vi "Actor Core.vi"(8 "error in":errorcluster, 11 "DUTMotor in":refnum<class "DUTMotor.lvclass">) -> (0 "error out":errorcluster, 3 "Actor out":refnum<class "Actor.lvclass">)   [LabVIEW 2024, in "DUTMotor Actor.lvlib" / "DUTMotor.lvclass"]
doc: "<p>(<strong>Filename</strong>: <span class=\"dnl\">Actor Framework.lvlib:Actor.lvclass:Actor Core.vi</span>)</p>\n<p>Receives messages to the actor, reacts to them, and initiates any error handling that may shut the actor down.</p>\n<p>Descendant classes may override this VI to append parallel tasks for the actor to complete while it handles messages. Overrides use the <a href=\"nihelplauncher://docs/csh?context=lvcore_glang_udclass\">Call Parent Class Method</a> node.</p>"
uses:
  DUTMotor.lvclass
  C:/Program Files (x86)/National Instruments/LabVIEW 2024/vi.lib/ActorFramework/Actor/Actor.lvclass
  <vilib>/ActorFramework/Actor/Actor.lvclass
  DUTMotor.lvclass/DUTMotor.ctl
  DUTMotorActFunc.ctl
  <vilib>/ActorFramework/Actor/Actor.lvclass/Actor.ctl
  MFActor/ActorMessage/MF Task Name.ctl
  MFActor/NestedActorName.ctl
  MFActor/DeviceAlias.ctl
  ref/PCANUSB/PCANUSB.lvclass
  MFActor/ActorMessage/MFActorMsg.lvclass
panel:
  out "UpdateData":bool
  out "Col Index Map":map{string, i32}(c390)
  out "MeasData":dbl[](array[numeric])
  out "In Query":bool
  out "Data":u8[](array[numeric])
  in  "EndProc":bool
  out "Connected":bool
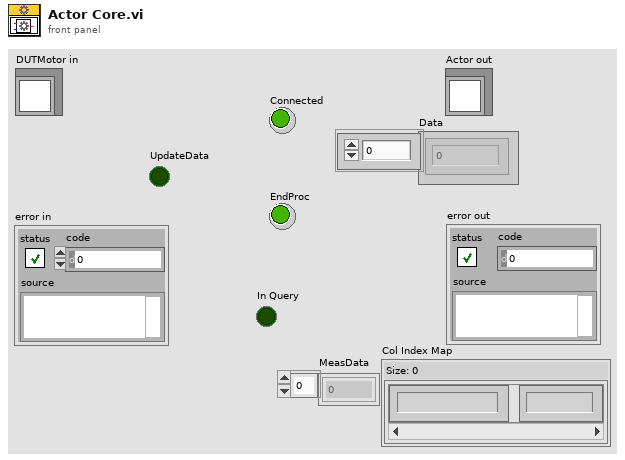
[diagram p1: front panel]
types:
  T1 = typedef "DUTMotorActFunc.ctl" = enum16{"None", "Config", "ConfigMeasData", "Query", "ConvertData", "End"}
  T2 = typedef "NestedActorName.ctl" = enum16{"None", "4503#0", "4503#1", "AIO#0", "AIO#1", "DIO", "PID", "TCPIP", "TestAngle", "TestFixPt", "TestMultiPt", "TestSinWave", "PW3390", "ADAM4118", "DUT Motor"}
  T3 = typedef "MF Task Name.ctl" = enum16{"DIChanged", "UpdateErrorCode", "SetTorque", "SetDriveTorque", "DataUpdated", "RunningTestProc", "StreamCtrl", "RunPID", "StopTest", "TCP Conn", "RefreshAutoUI", "ZeroAngle", "NestedActorLaunched", "NestedActorEnded", "ShowPsMsg"}
  T4 = typedef "DeviceAlias.ctl" = enum16{"TQM0", "TQM1", "PM", "THERMO", "DC POWER", "DUT Motor"}
  T5 = cluster{"message_id":i32, "CAN Signals":cluster{"signal_name":string, "start_bit":i32, "length":i32, "byte_order":string, "sign":string, "factor":dbl, "offset":dbl, "unit":string}[]}[]
  T6 = cluster{"message_id":i32, "CAN Signals":cluster{"signal_name":string, "start_bit":i32, "length":i32, "byte_order":string, "sign":string, "factor":dbl, "offset":dbl, "unit":string}[]}
  T7 = cluster{"signal_name":string, "start_bit":i32, "length":i32, "byte_order":string, "sign":string, "factor":dbl, "offset":dbl, "unit":string}[]
  T8 = cluster{"MF Msg Enum":T3, cluster{"MeasData":dbl[], "Device":T4}}
  T9 = cluster{"DUTMotorActFunc":T1, "ConfigMeasData":string[]}
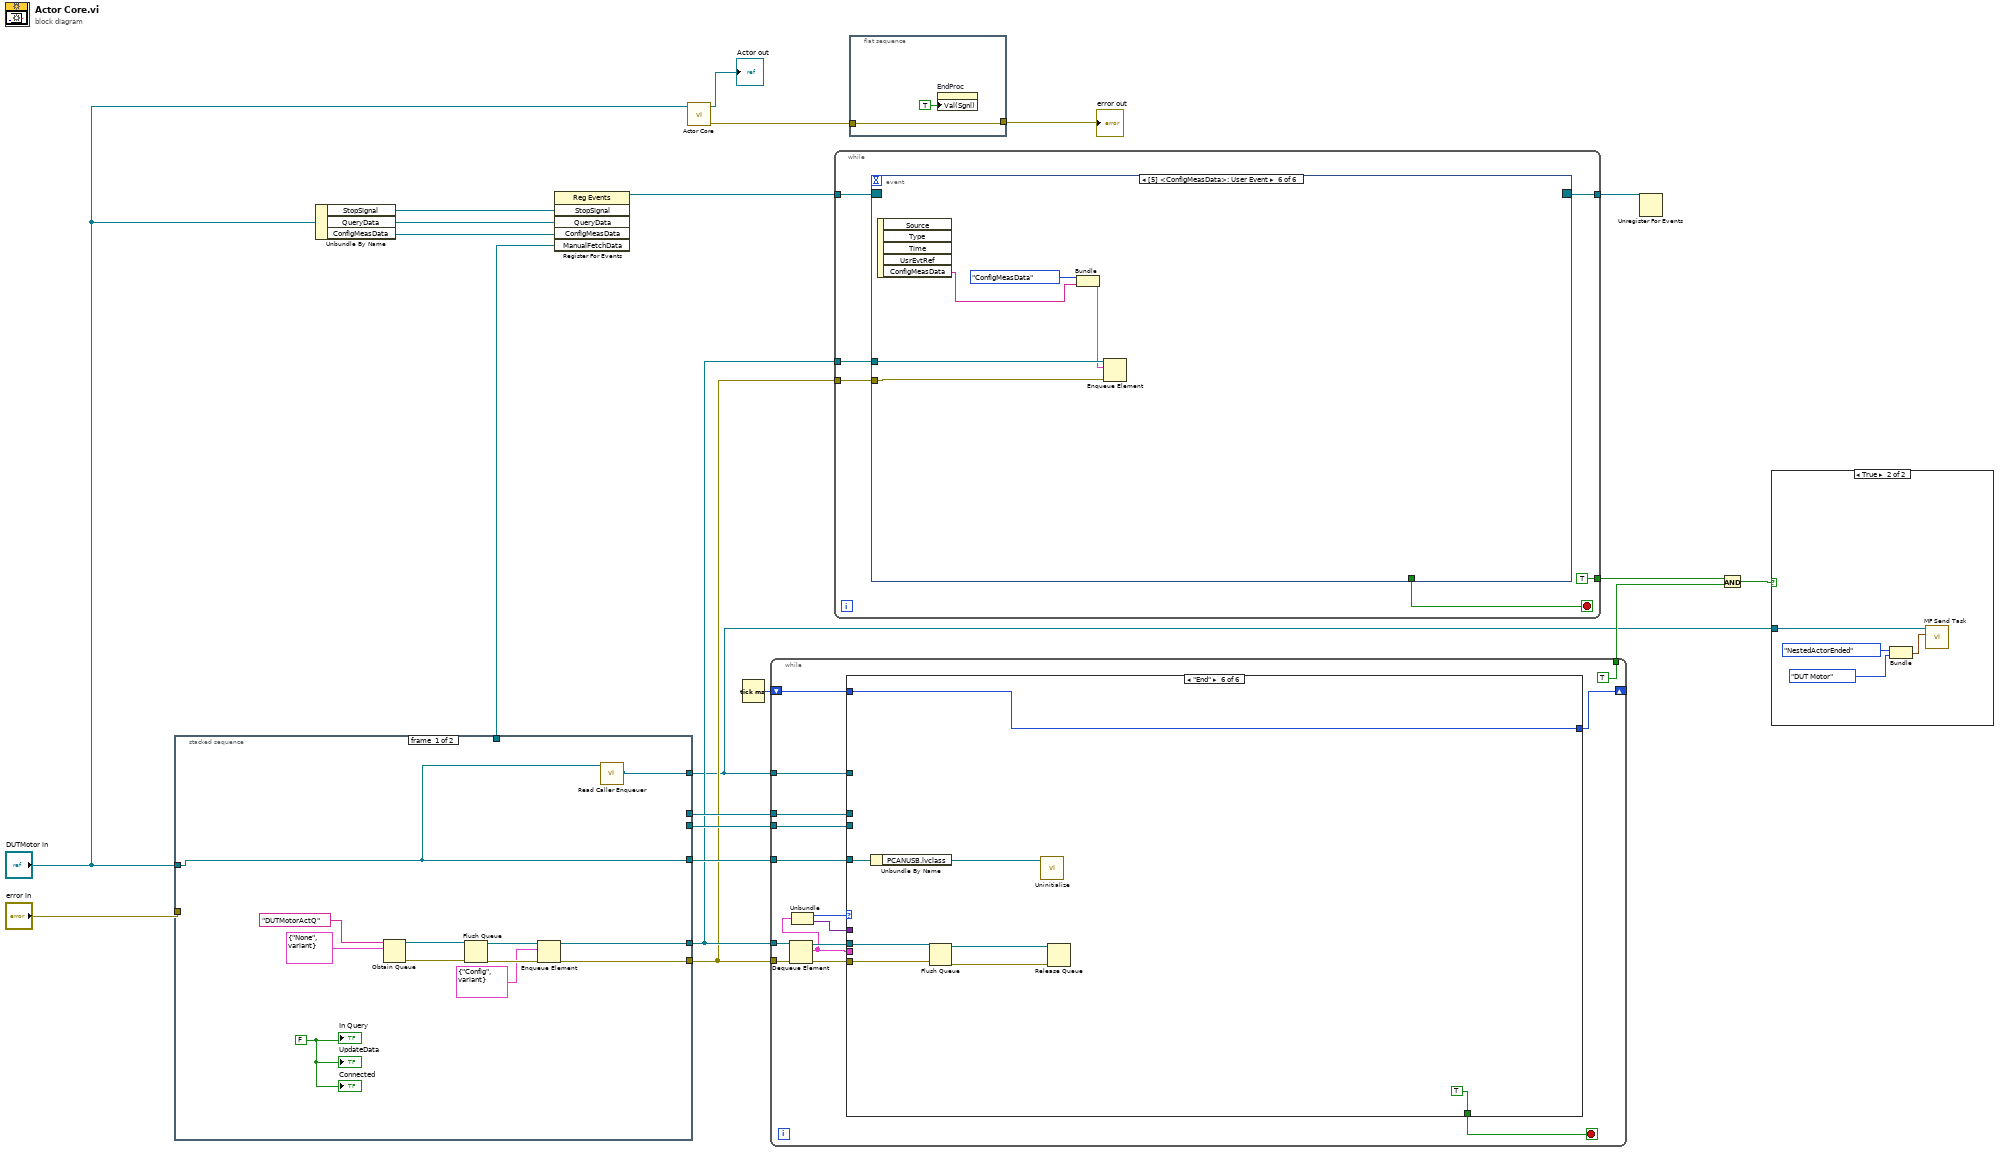
[diagram p0: block diagram]
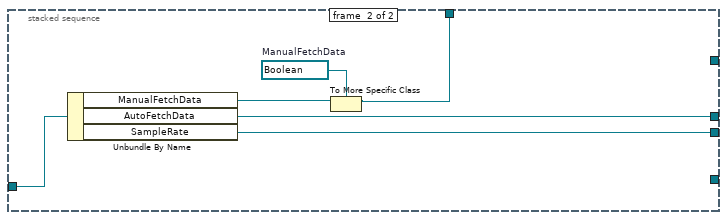
[diagram p3: hidden frame]
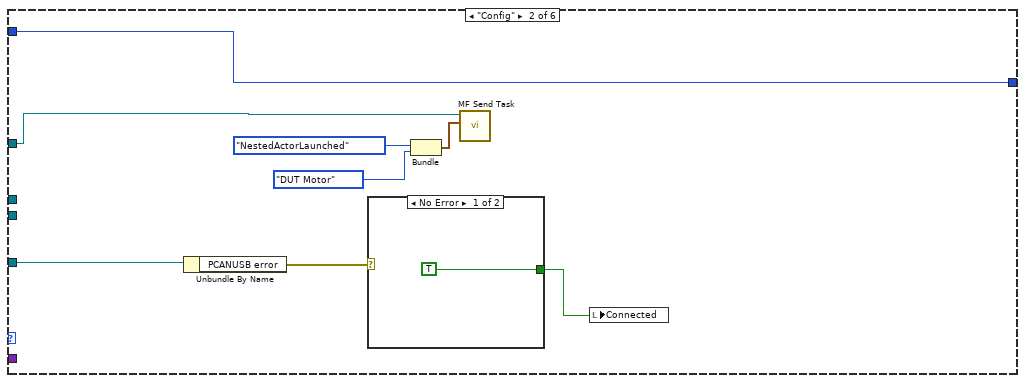
[diagram p5: hidden frame]
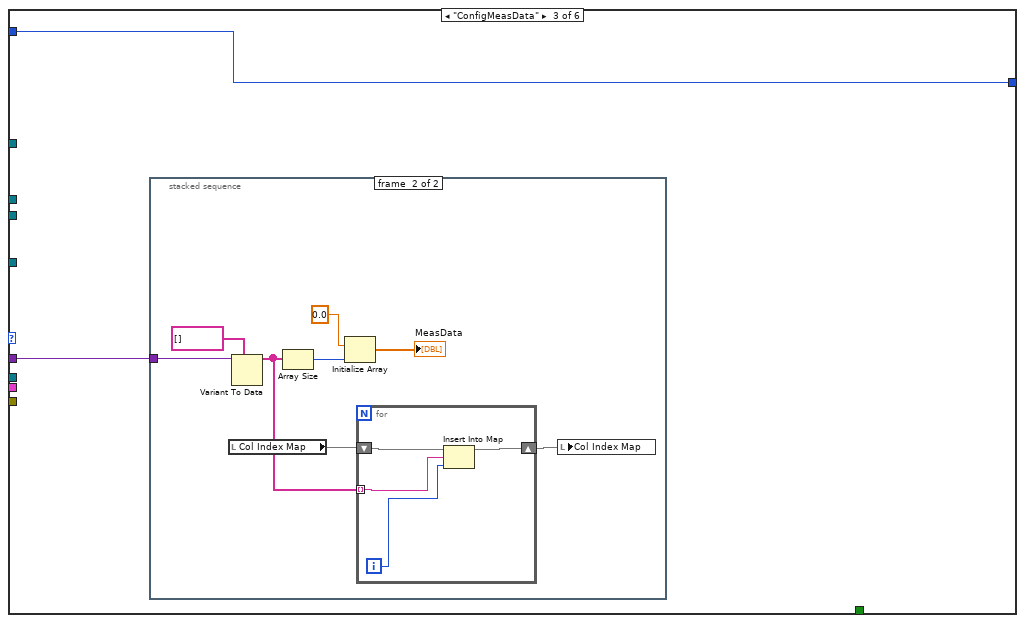
[diagram p7: hidden frame]
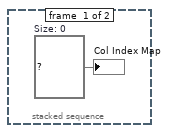
[diagram p8: hidden frame]
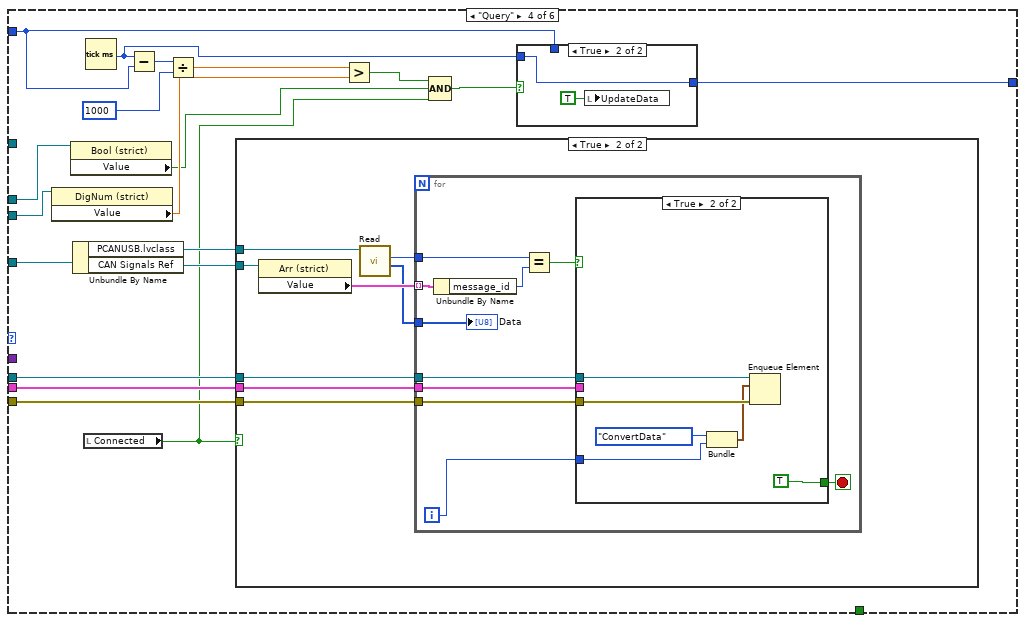
[diagram p9: hidden frame]
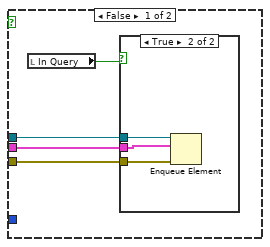
[diagram p12: hidden frame]
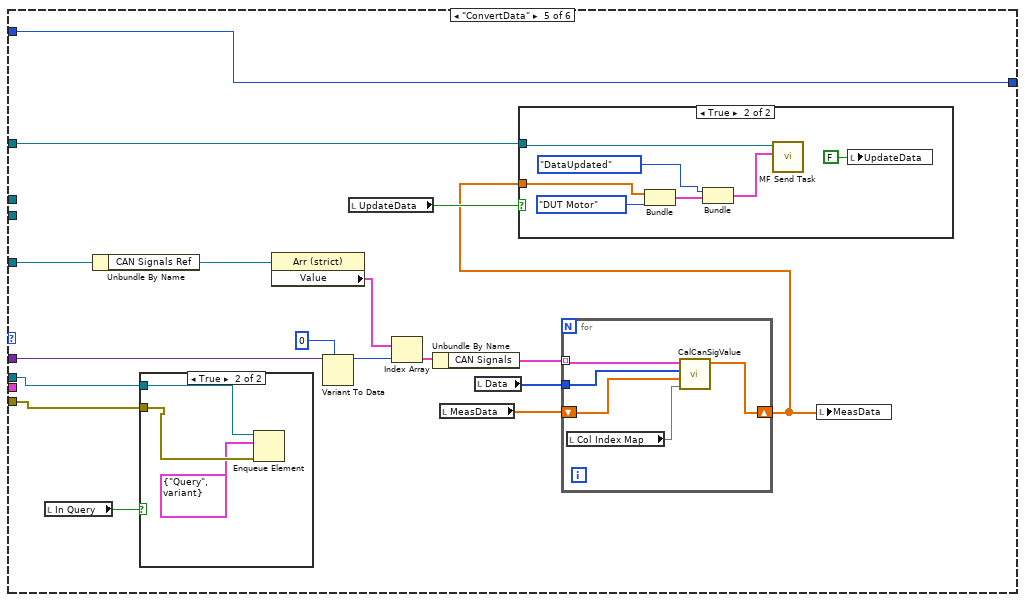
[diagram p14: hidden frame]
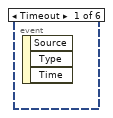
[diagram p17: hidden frame]
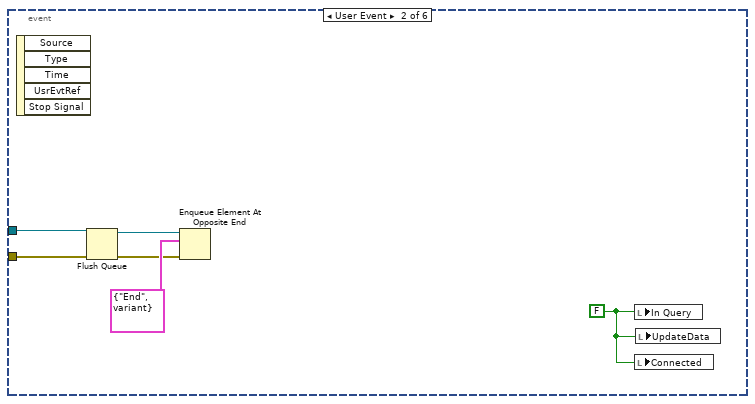
[diagram p18: hidden frame]
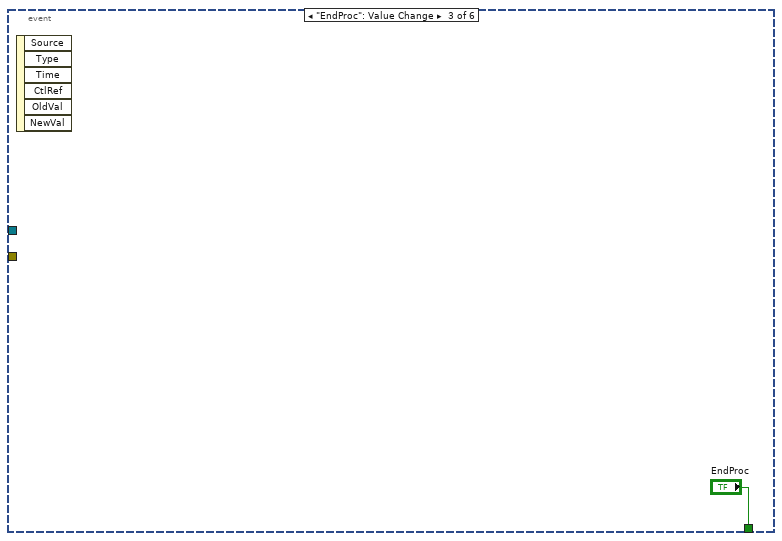
[diagram p19: hidden frame]
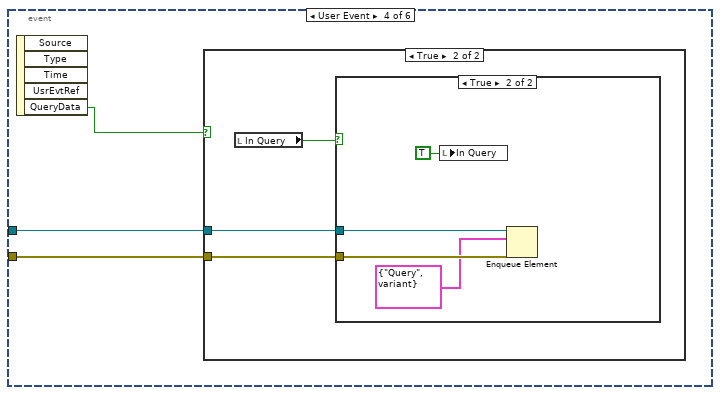
[diagram p20: hidden frame]
diagram:
  n1 = stacked-sequence {
    tunnel: "error in" -> [_ _]
    tunnel: "DUTMotor in" -> [w24 w39]
    tunnel: [w26 _] -> w9
    tunnel: [w25 _] -> w8
    tunnel: [w24 _] -> w19
    tunnel: [_ w38] -> w18
    tunnel: [_ w37] -> w17
    tunnel: [_ w34] -> w11
    tunnel: [w23 _] -> w2
    frame #0 {
      w22 = FALSE
      n2 = Obtain Queue(name (unnamed)="DUTMotorActQ", element data type=cluster{"DUTMotorActFunc":T1, variant} {"DUTMotorActFunc"=enum."None", variant}) -> (queue out=w31:refnum<queue>, error out=w30:errorcluster)  [unwired: 3 in, 1 out]
      n3 = Flush Queue(queue=w31, error in (no error)=w30) -> (queue out=w29:refnum<queue>, error out=w28:errorcluster)  [unwired: 1 out]
      n4 = Enqueue Element(queue=w29, element=cluster{"DUTMotorActFunc":T1, variant} {"DUTMotorActFunc"=enum."Config", variant}, error in (no error)=w28) -> (queue out=w26:refnum<queue>, error out=w25:errorcluster)  [unwired: 1 in, 1 out]
      n5 = call <vilib>:"Read Caller Enqueuer.vi"("Actor"=w24) -> ("Caller Enqueuer"=w23:refnum<class "Message Enqueuer.lvclass">)  [unwired: 10 in]
      "In Query" <- w22
      "UpdateData" <- w22
      "Connected" <- w22
    }
    frame #1 {
      w35 = refnum<vi> refnum  # ManualFetchData
      n6 = Unbundle By Name(w39) -> ("ManualFetchData"=w36:refnum<vi>, "AutoFetchData"=w38:refnum<vi>, "SampleRate"=w37:refnum<vi>)
      n7 = To More Specific Class(target class=w35, reference=w36) -> (specific class reference=w34:refnum<vi>)  [unwired: 1 in, 1 out]
    }
  }
  n8 = Unbundle By Name("DUTMotor in") -> ("StopSignal"=w14:refnum<user-event>, "QueryData"=w13:refnum<user-event>, "ConfigMeasData"=w1:refnum<user-event>)
  n9 = register-events(w14, w13, w1, w11) -> (reference out=w12:refnum<event-registration>)  [unwired: 2 in, 1 out]
  n10 = call-parent "Actor Core.vi"("Actor in"="DUTMotor in") -> ("error out"=w7:errorcluster, "Actor out"=→"Actor out":refnum<class "Actor.lvclass">)  [unwired: 9 in]
  n11 = Tick Count (ms)() -> (millisecond timer value=w16:u32)
  n12 = while {
    tunnel: w9 -> [w54]
    tunnel: w8 -> [w53]
    tunnel: w19 -> [w48]
    tunnel: w18 -> [w47]
    tunnel: w17 -> [w46]
    shift-right: [w43] -> _
    shift-left: w16 -> [w44]
    tunnel: w2 -> [w41]
    tunnel: [TRUE] -> w4
    stop <- w45 stop-if-true
    n13 = Dequeue Element(queue=w54, error in (no error)=w53) -> (queue out=w52:refnum<queue>, element=w42:cluster{"DUTMotorActFunc":T1, variant}, error out=w51:errorcluster)  [unwired: 1 in, 1 out]
    n14 = Unbundle(w42) -> ("DUTMotorActFunc"=w50:T1, w49:variant)
    n15 = case shown="\"End\"" w50 {
      tunnel: w52 -> [_ _ _ w95 w134 w172]
      tunnel: w51 -> [_ _ _ w94 w133 w171]
      tunnel: w49 -> [_ _ w66 _ w148 _]
      tunnel: w48 -> [_ w63 _ w98 w146 w166]
      tunnel: w47 -> [_ _ _ w92 _ _]
      tunnel: w46 -> [_ _ _ w91 _ _]
      tunnel: [_ _ _ _ _ TRUE] -> w45
      tunnel: [w55 w61 w65 w80 w149 w167] -> w43
      tunnel: w44 -> [w55 w61 w65 w81 w149 w167]
      tunnel: w42 -> [_ _ _ w93 _ _]
      tunnel: w41 -> [_ w57 _ _ w137 _]
      frame "None", Default {
      }
      frame "Config" {
        n16 = Unbundle By Name(w63) -> ("PCANUSB error"=w62:errorcluster)
        n17 = case shown="No Error" w62 {
          tunnel: [TRUE _] -> w56
          frame No Error {
          }
          frame Error {
          }
        }
        n18 = Bundle("MF Msg Enum"=MF_Task_Name."NestedActorLaunched", "NestedActorName"=NestedActorName."DUT Motor") -> (w60:cluster{"MF Msg Enum":T3, "NestedActorName":T2})  [unwired: 1 in]
        n19 = call "MF Send Task.vi"("MsgType"=w60, "Message Enqueuer"=w57) -> ()  [unwired: 9 in, 1 out]
        n20 = local write "Connected"(w56) -> ()
      }
      frame "ConfigMeasData" {
        n21 = stacked-sequence {
          tunnel: w66 -> [_ w75]
          frame #0 {
            w67 = map{string, i32} {}  # Size: 0
            "Col Index Map" <- w67
          }
          frame #1 {
            n22 = local read "Col Index Map"() -> (w69:map{string, i32})
            n23 = Variant To Data(type=string[] [], Variant=w75) -> (data=w70:string[])  [unwired: 1 in, 1 out]
            n24 = Array Size(array=w70) -> (size(s)=w73:i32)
            n25 = Initialize Array(0.0, w73) -> (→"MeasData":dbl[])
            n26 = for {
              tunnel: w70 -> [w78] mode=indexing
              shift-right: [w76] -> w68
              shift-left: w69 -> [w79]
              i -> [w77]
              n27 = Insert Into Map(map in=w79, key=w78, value=w77) -> (map out=w76:map{string, i32})  [unwired: 2 out]
            }
            n28 = local write "Col Index Map"(w68) -> ()
          }
        }
      }
      frame "Query" {
        n29 = property class="DigNum (strict)"(reference=w91) -> ("Value"=w87:dbl)  [unwired: 1 in, 2 out]
        n30 = property class="Bool (strict)"(reference=w92) -> ("Value"=w85:bool)  [unwired: 1 in, 2 out]
        n31 = Unbundle By Name(w98) -> ("PCANUSB.lvclass"=w96:refnum<class "PCANUSB.lvclass">, "CAN Signals Ref"=w97:refnum<vi>)
        n32 = local read "Connected"() -> (w84:bool)
        n33 = Tick Count (ms)() -> (millisecond timer value=w82:u32)
        n34 = Subtract(x=w82, y=w81) -> (x-y=w90:u32)
        n35 = Divide(x=w90, y=u32 1000) -> (x/y=w88:dbl)
        n36 = case shown="True" w84 {
          tunnel: w97 -> [_ w109]
          tunnel: w96 -> [_ w108]
          tunnel: w95 -> [_ w104]
          tunnel: w94 -> [_ w103]
          tunnel: w93 -> [_ w102]
          frame False {
          }
          frame True {
            n37 = property class="Arr (strict)"(reference=w109) -> ("Value"=w107:T5)  [unwired: 1 in, 2 out]
            n38 = call "Read.vi"("PCANUSB in"=w108) -> ("Data"=w105:u8[], "ID"=w106:u32)  [unwired: 5 in, 4 out]
            n39 = for {
              tunnel: w107 -> [w119] mode=indexing
              tunnel: w106 -> [w117]
              tunnel: w105 -> [w114]
              tunnel: w104 -> [w113]
              tunnel: w103 -> [w112]
              tunnel: w102 -> [w110]
              i -> [w111]
              stop <- w115 stop-if-true
              n40 = Unbundle By Name(w119) -> ("message_id"=w118:i32)
              n41 = Equal?(x=w117, y=w118) -> (x = y?=w116:bool)
              n42 = case shown="True" w116 {
                tunnel: [_ TRUE] -> w115
                tunnel: w113 -> [w122 w131]
                tunnel: w112 -> [w121 w130]
                tunnel: w111 -> [_ w128]
                tunnel: w110 -> [w120 _]
                frame False {
                  n43 = local read "In Query"() -> (w123:bool)
                  n44 = case shown="True" w123 {
                    tunnel: w122 -> [_ w126]
                    tunnel: w121 -> [_ w125]
                    tunnel: w120 -> [_ w124]
                    frame False {
                    }
                    frame True {
                      n45 = Enqueue Element(queue=w126, element=w124, error in (no error)=w125) -> ()  [unwired: 1 in, 3 out]
                    }
                  }
                }
                frame True {
                  n46 = Bundle("DUTMotorActFunc"=DUTMotorActFunc."ConvertData", w128) -> (w127:cluster{"DUTMotorActFunc":T1, i32})  [unwired: 1 in]
                  n47 = Enqueue Element(queue=w131, element=w127, error in (no error)=w130) -> ()  [unwired: 1 in, 3 out]
                }
              }
              "Data" <- w114
            }
          }
        }
        n48 = Greater?(x=w88, y=w87) -> (0:w86:bool)
        n49 = Compound Arithmetic op=AND(w86, w85, w84) -> (w83:bool)
        n50 = case shown="True" w83 {
          tunnel: w82 -> [_ w101]
          tunnel: [w99 w101] -> w80
          tunnel: w81 -> [w99 _]
          frame False {
          }
          frame True {
            n51 = local write "UpdateData"(TRUE ("UpdateData")) -> ()
          }
        }
      }
      frame "ConvertData" {
        n52 = local read "In Query"() -> (w135:bool)
        n53 = Unbundle By Name(w146) -> ("CAN Signals Ref"=w145:refnum<vi>)
        n54 = case shown="True" w135 {
          tunnel: w134 -> [_ w152]
          tunnel: w133 -> [_ w151]
          frame False {
          }
          frame True {
            n55 = Enqueue Element(queue=w152, element=cluster{"DUTMotorActFunc":T1, variant} {"DUTMotorActFunc"=enum."Query", variant}, error in (no error)=w151) -> ()  [unwired: 1 in, 3 out]
          }
        }
        n56 = property class="Arr (strict)"(reference=w145) -> ("Value"=w144:T5)  [unwired: 1 in, 2 out]
        n57 = Variant To Data(type=0, Variant=w148) -> (data=w143:i32)  [unwired: 1 in, 1 out]
        n58 = local read "UpdateData"() -> (w138:bool)
        n59 = Index Array(array=w144, index=w143) -> (element=w142:T6)
        n60 = Unbundle By Name(w142) -> ("CAN Signals"=w141:T7)
        n61 = local read "MeasData"() -> (w139:dbl[])
        n62 = local read "Data"() -> (w140:u8[])
        n63 = for {
          tunnel: w141 -> [w164] mode=indexing
          tunnel: w140 -> [w163]
          shift-right: [w161] -> w136
          shift-left: w139 -> [w162]
          n64 = local read "Col Index Map"() -> (w160:map{string, i32})
          n65 = call "CalCanSigValue.vi"("Col Index Map"=w160, "MeasData"=w162, "RawData"=w163, "SignalFormat"=w164) -> ("MeasData.out"=w161:dbl[])  [unwired: 7 in]
        }
        n66 = case shown="True" w138 {
          tunnel: w137 -> [_ w158]
          tunnel: w136 -> [_ w153]
          frame False {
          }
          frame True {
            n67 = Bundle("MeasData"=w153, "Device"=DeviceAlias."DUT Motor") -> (w155:cluster{"MeasData":dbl[], "Device":T4})  [unwired: 1 in]
            n68 = Bundle("MF Msg Enum"=MF_Task_Name."DataUpdated", w155) -> (w154:T8)  [unwired: 1 in]
            n69 = call "MF Send Task.vi"("MsgType"=w154, "Message Enqueuer"=w158) -> ()  [unwired: 9 in, 1 out]
            n70 = local write "UpdateData"(FALSE ("UpdateData")) -> ()
          }
        }
        n71 = local write "MeasData"(w136) -> ()
      }
      frame "End" {
        n72 = Unbundle By Name(w166) -> ("PCANUSB.lvclass"=w165:refnum<class "PCANUSB.lvclass">)
        n73 = Flush Queue(queue=w172, error in (no error)=w171) -> (queue out=w170:refnum<queue>, error out=w169:errorcluster)  [unwired: 1 out]
        n74 = call "Uninitialize.vi"("PCANUSB in"=w165) -> ()  [unwired: 9 in, 2 out]
        n75 = Release Queue(queue=w170, error in (no error)=w169) -> ()  [unwired: 1 in, 3 out]
      }
    }
  }
  n76 = while {
    tunnel: w12 -> [w178]
    tunnel: [w177] -> w10
    tunnel: w9 -> [w176]
    tunnel: w8 -> [w175]
    tunnel: [TRUE] -> w5
    stop <- w174 stop-if-true
    n77 = event shown="[5] <ConfigMeasData>: User Event" {
      selector: w178 -> [_ _ _ _ _ _]
      dyn-events: [_ _ _ _ _ _] -> w177
      timeout: _ -> [_ _ _ _ _ _]
      tunnel: w176 -> [_ w183 _ w187 _ w202]
      tunnel: w175 -> [_ w182 _ w186 _ w201]
      tunnel: [_ _ "EndProc" _ _ _] -> w174
      event Timeout {
        n78 = event-data() -> ()  [unwired: 1 in, 3 out]
      }
      event User Event {
        w179 = FALSE
        n79 = event-data() -> ()  [unwired: 1 in, 5 out]
        n80 = Flush Queue(queue=w183, error in (no error)=w182) -> (queue out=w181:refnum<queue>, error out=w180:errorcluster)  [unwired: 1 out]
        n81 = Enqueue Element At Opposite End(queue=w181, element=cluster{"DUTMotorActFunc":T1, variant} {"DUTMotorActFunc"=enum."End", variant}, error in (no error)=w180) -> ()  [unwired: 1 in, 3 out]
        n82 = local write "In Query"(w179) -> ()
        n83 = local write "Connected"(w179) -> ()
        n84 = local write "UpdateData"(w179) -> ()
      }
      event "EndProc": Value Change {
        n85 = event-data() -> ()  [unwired: 1 in, 6 out]
      }
      event User Event {
        n86 = event-data() -> ("QueryData"=w188:bool)  [unwired: 1 in, 4 out]
        n87 = case shown="True" w188 {
          tunnel: w187 -> [_ w191]
          tunnel: w186 -> [_ w190]
          frame False {
            n88 = local write "In Query"(FALSE ("In Query")) -> ()
          }
          frame True {
            n89 = local read "In Query"() -> (w192:bool)
            n90 = case shown="True" w192 {
              tunnel: w191 -> [_ w196]
              tunnel: w190 -> [_ w195]
              frame False {
              }
              frame True {
                n91 = local write "In Query"(TRUE ("In Query")) -> ()
                n92 = Enqueue Element(queue=w196, element=cluster{"DUTMotorActFunc":T1, variant} {"DUTMotorActFunc"=enum."Query", variant}, error in (no error)=w195) -> ()  [unwired: 1 in, 3 out]
              }
            }
          }
        }
      }
      event Value Change {
        n93 = event-data() -> ()  [unwired: 1 in, 6 out]
        n94 = local write "UpdateData"(TRUE ("UpdateData")) -> ()
      }
      event User Event {
        n95 = event-data() -> ("ConfigMeasData"=w199:string[])  [unwired: 1 in, 4 out]
        n96 = Bundle("DUTMotorActFunc"=DUTMotorActFunc."ConfigMeasData", "ConfigMeasData"=w199) -> (w198:T9)  [unwired: 1 in]
        n97 = Enqueue Element(queue=w202, element=w198, error in (no error)=w201) -> ()  [unwired: 1 in, 3 out]
      }
    }
  }
  n98 = flat-sequence {
    tunnel: w7 -> [w204]
    tunnel: [w204] -> w6
    frame #0 {
      n99 = property on="EndProc" class="Bool (strict)"("Val(Sgnl)"=TRUE ("Value (Signaling)")) -> ()  [unwired: 2 in, 2 out]
    }
  }
  n100 = Unregister For Events(event registration refnum=w10) -> ()  [unwired: 1 in, 1 out]
  n101 = Compound Arithmetic op=AND(w5, w4) -> (w3:bool)
  n102 = case shown="True" w3 {
    tunnel: w2 -> [_ w208]
    frame False {
    }
    frame True {
      n103 = Bundle("MF Msg Enum"=MF_Task_Name."NestedActorEnded", "NestedActorName"=NestedActorName."DUT Motor") -> (w205:cluster{"MF Msg Enum":T3, "NestedActorName":T2})  [unwired: 1 in]
      n104 = call "MF Send Task.vi"("MsgType"=w205, "Message Enqueuer"=w208) -> ()  [unwired: 9 in, 1 out]
    }
  }
  "error out" <- w6
